vi "Read.vi"(7 "I2C Channel (0)":u8, 8 "Error In":errorcluster, 11 "LINX Resource":T2) -> (0 "Error Out":errorcluster, 2 "Acceleration Data (g)":T1, 3 "LINX Resource":T2)   [LabVIEW 2020, in "LMH-LINX.lvlib" / "HiTechnic.lvlib" / "Accelerometer.lvlib"]
doc: "Read a single point of data containing the X, Y and Z axis of acceleration (in g) from the HiTechnic accelerometer."
uses:
  Accelerometer.lvlib
  Private/Type Defs/LINX Ref.ctl
  Private/Type Defs/Platform.ctl
  Private/Type Defs/Interface.ctl
  Private/Device/Type Defs/LINX Device Config.ctl
  Private/Device/Type Defs/TCP Config.ctl
  Private/Device/Type Defs/Channels.ctl
  Private/Local IO/LinxI2cWrite.vi
  Utilities/Check Channel.vi
  Private/Utilties/Generate Error.vi
  LMH-LINX.lvlib
  Private/Device/Device.lvlib
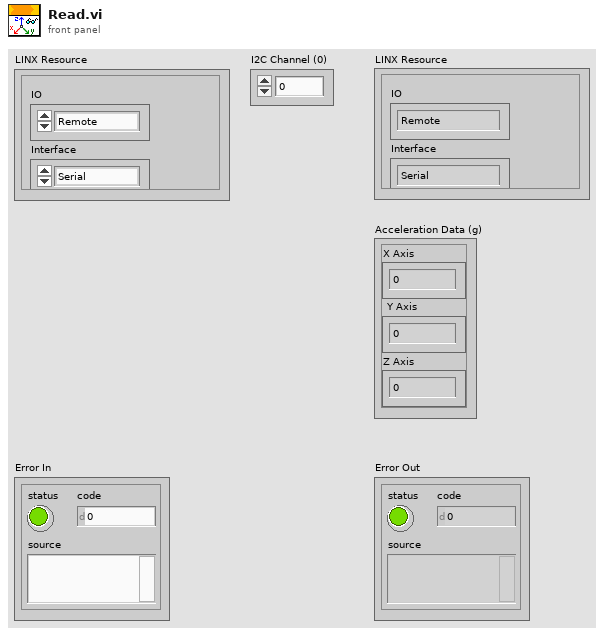
[diagram p1: front panel]
types:
  T1 = cluster{"X Axis":dbl, "Y Axis":dbl, "Z Axis":dbl}
  T2 = typedef "LMH-LINX.lvlib/LINX Ref.ctl" = cluster{"IO":T3, "Interface":T4, "LINX Device Config":T5}
  T3 = typedef "LMH-LINX.lvlib/Platform.ctl" = enum16{"Remote", "Local"}
  T4 = typedef "LMH-LINX.lvlib/Interface.ctl" = enum16{"Serial", "TCP"}
  T5 = typedef "LMH-LINX.lvlib/Device.lvlib/LINX Device Config.ctl" = cluster{"Interface":T4, "COM Port":refnum<visa-resource-name>, "TCP Configuration":T6, "Device Family":u8, "Device ID":u8, "Device Name":string, "TCP Ref":refnum<k5>, "Channels":T7}
  T6 = typedef "LMH-LINX.lvlib/Device.lvlib/TCP Config.ctl" = cluster{"IP Address":string, "Port":u16}
  T7 = typedef "LMH-LINX.lvlib/Channels.ctl" = cluster{"DI":u8[], "DO":u8[], "AI":u8[], "AO":u8[], "PWM":u8[], "QE":u8[], "UART":u8[], "I2C 2":u8[], "SPI":u8[], "CAN":u8[], "Servo":u8[], "AI Ref (V)":dbl, "AI Resolution (Bits)":u8, "AO Ref (V)":dbl, "AO Resolution (Bits)":u8}
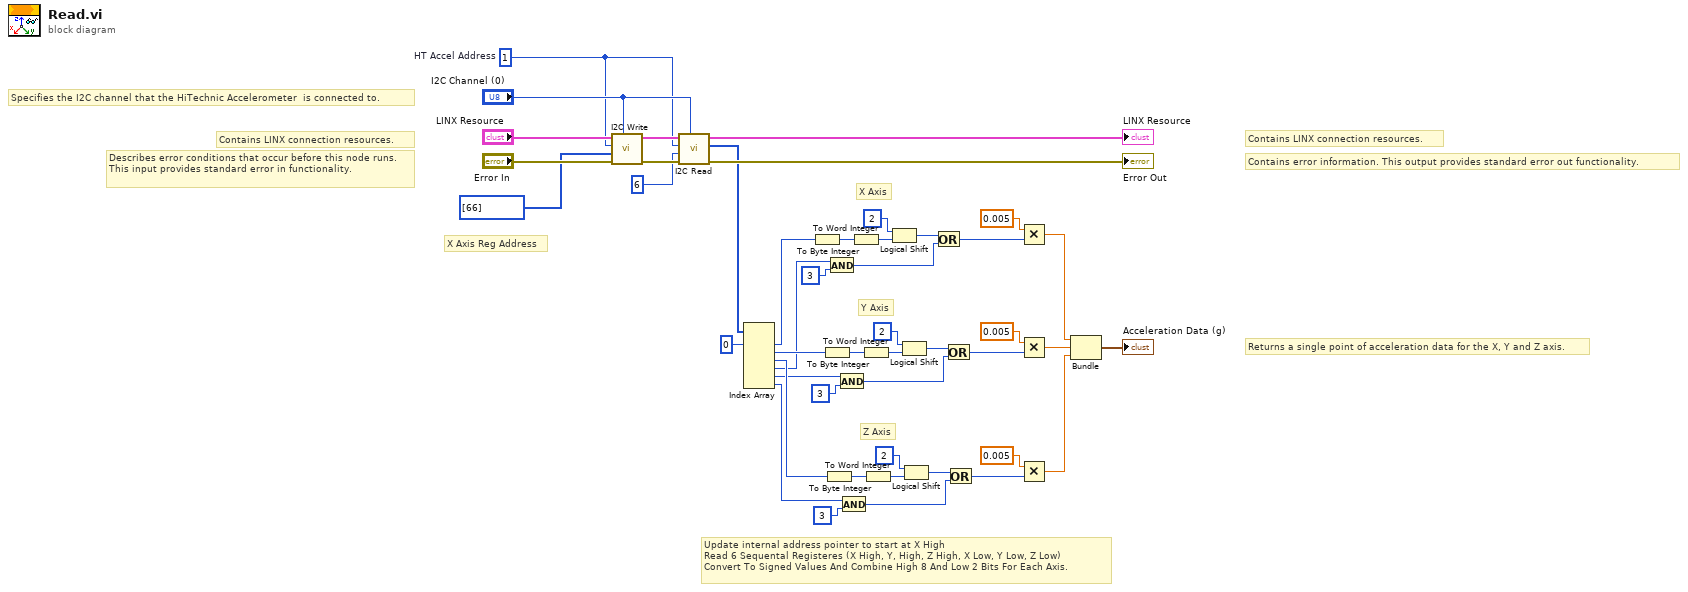
[diagram p0: block diagram]
diagram:
  w10 = u8 1  # HT Accel Address
  # "Returns a single point of acceleration data for the X, Y and Z axis."
  # "Contains LINX connection resources."
  # "Contains error information. This output provides standard error out functionality."
  # "Specifies the I2C channel that the HiTechnic Accelerometer  is connected to."
  # "Contains LINX connection resources."
  # "Describes error conditions that occur before this node runs. This input provides standard error in functionality."
  # "Update internal address pointer to start at X High\nRead 6 Sequental Registeres (X High, Y, High, Z High, X Low, Y Low, Z Low)\nConvert To Signed Values And Combine High 8 And Low 2 Bits For Each Axis."
  # "X Axis Reg Address"
  # "Z Axis"
  # "Y Axis"
  # "X Axis"
  n1 = call "I2C Write.vi"("I2C Channel"="I2C Channel (0)", "Error In"="Error In", "Data"=u8[] [66], "I2C Slave Address (0)"=w10, "LINX Resource"="LINX Resource") -> ("Error Out"=w46:errorcluster, "LINX Resource"=w45:T2)  [unwired: 5 in]
  n2 = call "I2C Read.vi"("I2C Channel"="I2C Channel (0)", "Error In"=w46, "Bytes To Read"=u8 6, "I2C Slave Address (0)"=w10, "LINX Resource"=w45) -> ("Error Out"=→"Error Out":errorcluster, "Data"=w8:u8[], "LINX Resource"=→"LINX Resource":T2)  [unwired: 4 in]
  n3 = Index Array(array=w8, index #1=0 ("index")) -> (element #1=w7:u8, element #2=w6:u8, element #3=w5:u8, element #4=w4:u8, element #5=w3:u8, element #6=w2:u8)  [unwired: 5 in]
  n4 = To Byte Integer(number=w7) -> (8bit integer=w31:i8)
  n5 = To Byte Integer(number=w6) -> (8bit integer=w26:i8)
  n6 = To Byte Integer(number=w5) -> (8bit integer=w15:i8)
  n7 = And(x=w4, y=i16 3) -> (x .and. y?=w34:i16)
  n8 = And(x=w3, y=i16 3) -> (x .and. y?=w25:i16)
  n9 = And(x=w2, y=i16 3) -> (x .and. y?=w16:i16)
  n10 = To Word Integer(number=w31) -> (16bit integer=w38:i16)
  n11 = To Word Integer(number=w26) -> (16bit integer=w21:i16)
  n12 = To Word Integer(number=w15) -> (16bit integer=w20:i16)
  n13 = Logical Shift(y=i16 2, x=w38) -> (x << y=w36:i16)
  n14 = Logical Shift(y=i16 2, x=w21) -> (x << y=w23:i16)
  n15 = Logical Shift(y=i16 2, x=w20) -> (x << y=w18:i16)
  n16 = Or(x=w36, y=w34) -> (x .or. y?=w32:i16)
  n17 = Or(x=w23, y=w25) -> (x .or. y?=w13:i16)
  n18 = Or(x=w18, y=w16) -> (x .or. y?=w14:i16)
  n19 = Multiply(x=0.005, y=w32) -> (x*y=w28:dbl)
  n20 = Multiply(x=0.005, y=w13) -> (x*y=w12:dbl)
  n21 = Multiply(x=0.005, y=w14) -> (x*y=w27:dbl)
  n22 = Bundle(w28, w12, w27) -> (→"Acceleration Data (g)":cluster{dbl, dbl, dbl})  [unwired: 1 in]
